vi "testPattern.vi"() -> ()   [LabVIEW 2011]
panel:
  out "Ramp Pattern":dbl[](array[numeric])
  in  "stop":bool
  in  "Image Pixels (Float)":sgl[][](array[numeric]) format="%.2f"
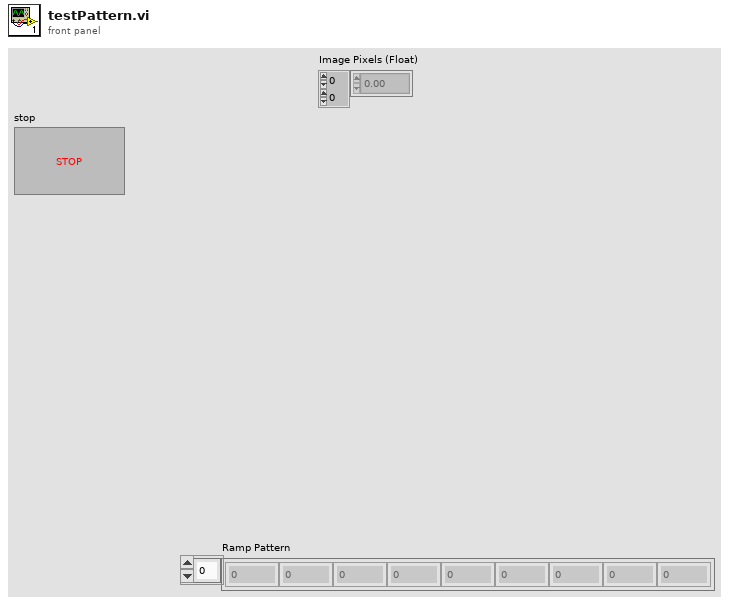
[diagram p1: front panel]
types:
  T1 = typedef "Image Type" = u32
  T2 = typedef "IMAQ Image.ctl" = refnum<image>
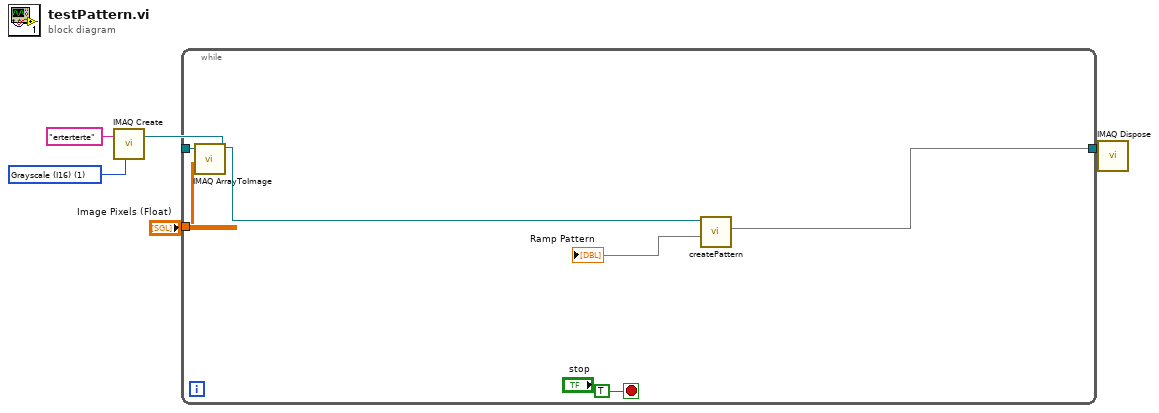
[diagram p0: block diagram]
diagram:
  w5 = T1 1 items=["Grayscale (U8)", "Grayscale (I16)", "Grayscale (SGL)", "Complex (CSG)", "RGB (U32)", "HSL (U32)", "RGB (U64)", "Grayscale (U16)"] ("Image Type")
  n1 = call "IMAQ Create"("Image Name"="erterterte", "Image Type"=w5) -> ("New Image"=w3:T2)  [unwired: 3 in, 1 out]
  n2 = while {
    tunnel: w3 -> [w11]
    tunnel: "Image Pixels (Float)" -> [w10]
    tunnel: [w9] -> w1
    stop <- TRUE stop-if-true
    n3 = call "IMAQ ArrayToImage"("Image Pixels (I16)"=w10, "Image"=w11) -> ("Image Out"=w8:T2)  [unwired: 8 in, 1 out]
    n4 = call "createPattern.vi"("Refnum in"=w8) -> (1:→"Ramp Pattern", 2:w9)  [unwired: 8 in, 1 out]
  }
  n5 = call "IMAQ Dispose"("Image"=w1) -> ()  [unwired: 5 in, 1 out]
